vi "Get Empty Cluster.vi"(8 "error in (no error)":errorcluster, 11 "Name":string) -> (0 "error out":errorcluster, 3 "Variant (Cluster) out":variant)   [LabVIEW 2017, in "Variant Data Manipulation.lvlib"]
uses:
  Variant Data Manipulation.lvlib
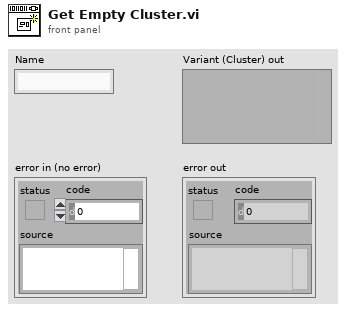
[diagram p1: front panel]
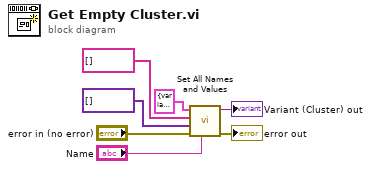
[diagram p0: block diagram]
diagram:
  n1 = call "Set All Names and Values.vi"("Cluster Name"="Name", "error in"="error in (no error)", "values"=variant[] [], "Element Names"=string[] [] ("Item Names"), "Cluster in"=cluster{variant} {variant}) -> ("error out"=→"error out":errorcluster, "Cluster out"=→"Variant (Cluster) out":variant)  [unwired: 5 in]
